vi "Remote Terminal Suite.vi"   [LabVIEW 2020, in "Unit Tests.lvlib"]
uses:
  Unit Tests.lvlib
  Tests/Remote Terminal/Remote Terminal.lvclass
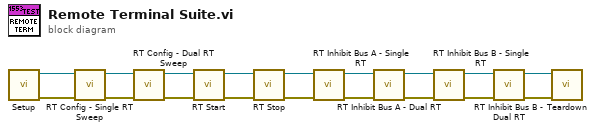
[diagram p0: block diagram]
diagram:
  n1 = call "Setup.vi"() -> ("error out"=w17:errorcluster, "1553 Unit Test out"=w18:refnum<class "Remote Terminal.lvclass">)  [unwired: 10 in]
  n2 = call "RT Config - Single RT Sweep.vi"("error in (no error)"=w17, "1553 Unit Test in"=w18) -> ("error out"=w2:errorcluster, "1553 Unit Test out"=w1:refnum<class "Remote Terminal.lvclass">)  [unwired: 8 in]
  n3 = call "RT Config - Dual RT Sweep.vi"("error in (no error)"=w2, "1553 Unit Test in"=w1) -> ("error out"=w6:errorcluster, "1553 Unit Test out"=w5:refnum<class "Remote Terminal.lvclass">)  [unwired: 8 in]
  n4 = call "RT Start.vi"("error in (no error)"=w6, "1553 Unit Test in"=w5) -> ("error out"=w4:errorcluster, "1553 Unit Test out"=w3:refnum<class "Remote Terminal.lvclass">)  [unwired: 8 in]
  n5 = call "RT Stop.vi"("error in (no error)"=w4, "1553 Unit Test in"=w3) -> ("error out"=w8:errorcluster, "1553 Unit Test out"=w7:refnum<class "Remote Terminal.lvclass">)  [unwired: 8 in]
  n6 = call "RT Inhibit Bus A - Single RT.vi"("error in (no error)"=w8, "1553 Unit Test in"=w7) -> ("error out"=w10:errorcluster, "1553 Unit Test out"=w9:refnum<class "Remote Terminal.lvclass">)  [unwired: 8 in]
  n7 = call "RT Inhibit Bus A - Dual RT.vi"("error in (no error)"=w10, "1553 Unit Test in"=w9) -> ("error out"=w14:errorcluster, "1553 Unit Test out"=w13:refnum<class "Remote Terminal.lvclass">)  [unwired: 8 in]
  n8 = call "RT Inhibit Bus B - Single RT.vi"("error in (no error)"=w14, "1553 Unit Test in"=w13) -> ("error out"=w12:errorcluster, "1553 Unit Test out"=w11:refnum<class "Remote Terminal.lvclass">)  [unwired: 8 in]
  n9 = call "RT Inhibit Bus B - Dual RT.vi"("error in (no error)"=w12, "1553 Unit Test in"=w11) -> ("error out"=w16:errorcluster, "1553 Unit Test out"=w15:refnum<class "Remote Terminal.lvclass">)  [unwired: 8 in]
  n10 = call "Teardown.vi"("error in (no error)"=w16, "1553 Unit Test in"=w15) -> ()  [unwired: 9 in, 1 out]
